vi "Get SMO HELP.vi"(8 "error in (no error)":errorcluster, 10 "Command":string, 11 "Inst.Transport in":refnum<class "Inst.Transport.lvclass">) -> (0 "error out":errorcluster, 2 "output cluster":T1, 3 "Inst.Transport out":refnum<class "Inst.Transport.lvclass">)   [LabVIEW 2019, in "Inst.Transport.lvclass"]
uses:
  Inst.Transport.lvclass
  <userlib>/LevyLab/Instrument Framework/subsystems/Help/typedefs/Help--cluster.ctl
  Typedefs/Inst.Transport.PublicCommands--Enum.ctl
  Typedefs/startTransport--Request--Cluster.ctl
  Typedefs/Inst.Transport.Methods--Enum.ctl
  Typedefs/getStatus--Reply--Cluster.ctl
  Typedefs/Inst.Transport.Status--Enum.ctl
  Typedefs/setExptFolder--Request--Cluster.ctl
  Typedefs/setExptComments--Request--Cluster.ctl
  Typedefs/setExptParam--Request--Cluster.ctl
  <userlib>/LevyLab/LV-Data/LV-Data/Typedefs/Dictionary--cluster.ctl
  Typedefs/setSweepConfig--Request--Cluster.ctl
  <userlib>/LevyLab/Lockin-Multichannel/Instrument.DAQ/Typedefs/Sweep.Channel--Cluster--Array.ctl
  <userlib>/LevyLab/Lockin-Multichannel/Instrument.DAQ/Typedefs/Sweep.Channel--Cluster.ctl
  <userlib>/LevyLab/Lockin-Multichannel/Instrument.DAQ/Typedefs/Sweep.Pattern--Enum.ctl
  <userlib>/LevyLab/Instrument Framework/Instrument Types/SCPI/Instrument.SCPI.lvclass
  <userlib>/LevyLab/Instrument Framework/subsystems/Help/Help.lvclass
  <userlib>/LevyLab/LV-Data/LV-Data/LV-Data.lvclass
  <userlib>/LevyLab/Lockin-Multichannel/Instrument.DAQ/Instrument.DAQ.lvclass
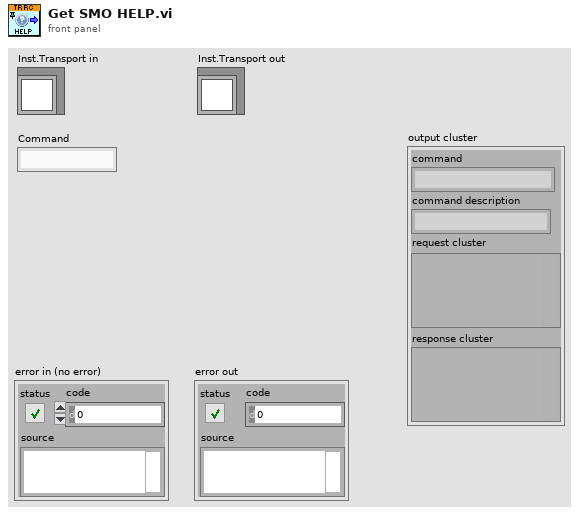
[diagram p1: front panel]
types:
  T1 = typedef "Instrument.lvlib/Help.lvclass/Help--cluster.ctl" = cluster{"command":string, "command description":string, "request cluster":variant, "response cluster":variant}
  T2 = typedef "Inst.Transport.lvclass/Inst.Transport.PublicCommands--Enum.ctl" = enum16{"startTransport", "stopTransport", "getStatus", "setExptFolder", "setExptComments", "appendExptParam", "clearExptParam", "setExptParam", "setSweepConfig"}
  T3 = typedef "Inst.Transport.lvclass/startTransport--Request--Cluster.ctl" = cluster{"method":T4}
  T4 = typedef "Inst.Transport.lvclass/Inst.Transport.Methods--Enum.ctl" = enum16{"LockinSweep", "LockinTime", "LockinTimeDelay"}
  T5 = typedef "Inst.Transport.lvclass/getStatus--Reply--Cluster.ctl" = cluster{"Status":T6}
  T6 = typedef "Inst.Transport.lvclass/Inst.Transport.Status--Enum.ctl" = enum16{"idle", "running"}
  T7 = typedef "Inst.Transport.lvclass/setExptFolder--Request--Cluster.ctl" = cluster{"folder":string}
  T8 = typedef "Inst.Transport.lvclass/setExptComments--Request--Cluster.ctl" = cluster{"comments":string}
  T9 = typedef "Inst.Transport.lvclass/setExptParam--Request--Cluster.ctl" = cluster{"param":T10}
  T10 = typedef "LV-Data.lvclass/Dictionary--cluster.ctl" = cluster{"key":string, "value":variant}
  T11 = typedef "Inst.Transport.lvclass/setSweepConfig--Request--Cluster.ctl" = cluster{"sweepTime":dbl, "initialWaitTime":dbl, "returnToStart":bool, "sweepChannels":T12}
  T12 = typedef "Instrument.Lockin.lvlib/Instrument.DAQ.lvclass/Sweep.Channel--Cluster--Array.ctl" = T13[]
  T13 = typedef "Instrument.Lockin.lvlib/Instrument.DAQ.lvclass/Sweep.Channel--Cluster.ctl" = cluster{"Enable?":bool, "Channel":u16, "Start":dbl, "End":dbl, "Pattern":T14, "Table":dbl[]}
  T14 = typedef "Instrument.Lockin.lvlib/Instrument.DAQ.lvclass/Sweep.Pattern--Enum.ctl" = enum16{"Ramp /", "Ramp /\\", "Smooth Ramp _/", "Smooth Ramp _/\\_", "Table"}
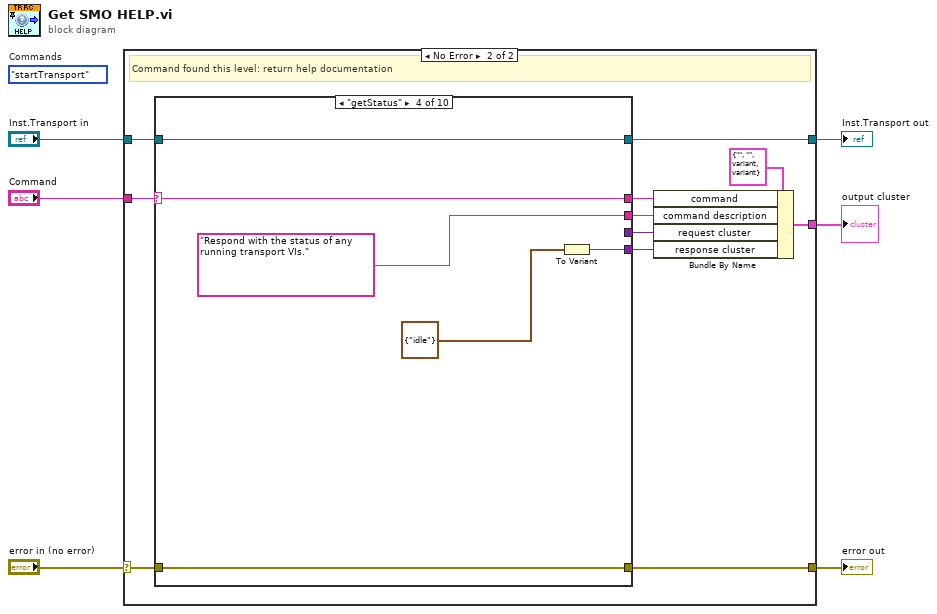
[diagram p0: block diagram]
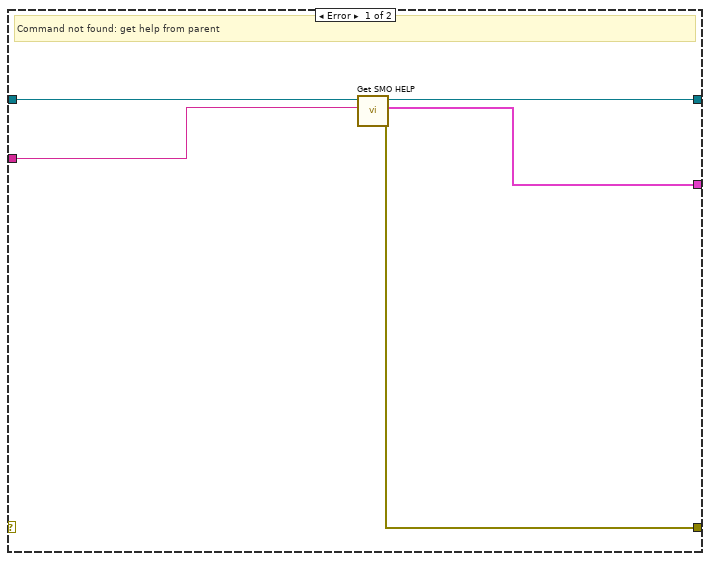
[diagram p2: hidden frame]
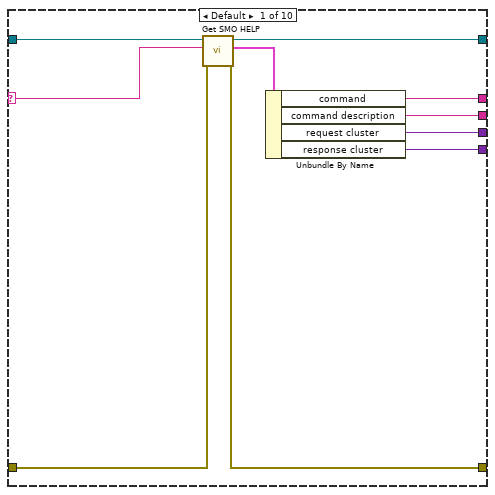
[diagram p3: hidden frame]
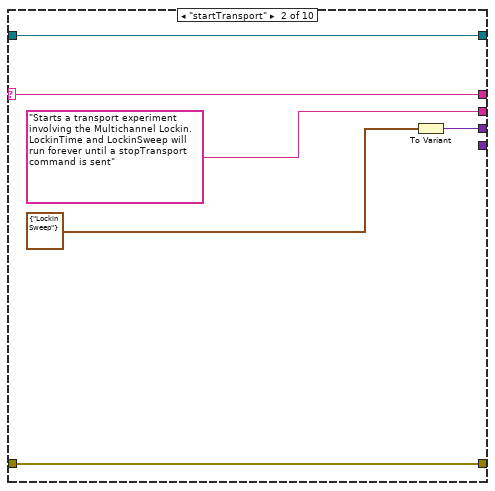
[diagram p4: hidden frame]
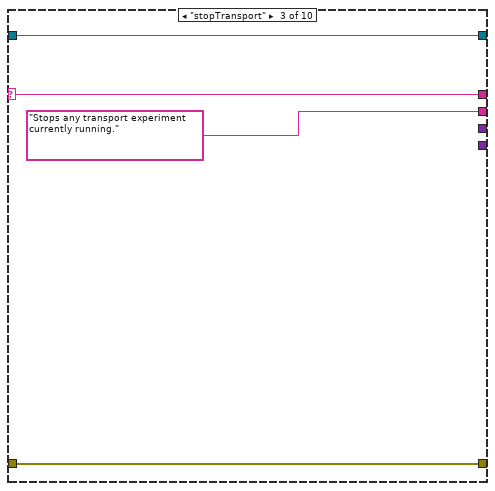
[diagram p5: hidden frame]
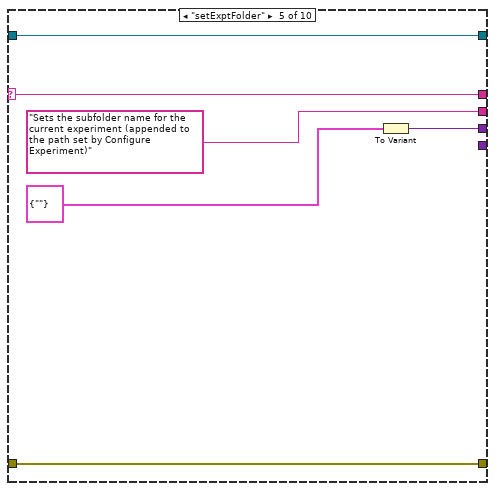
[diagram p6: hidden frame]
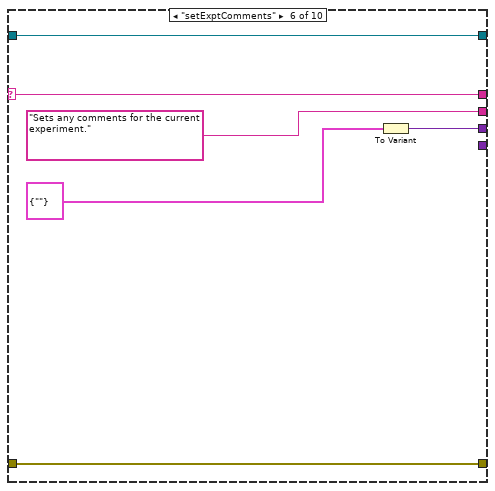
[diagram p7: hidden frame]
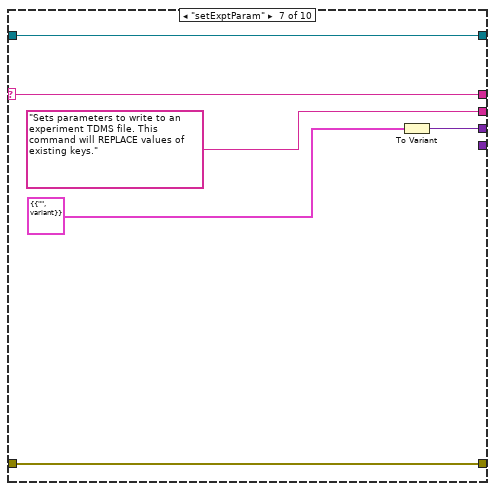
[diagram p8: hidden frame]
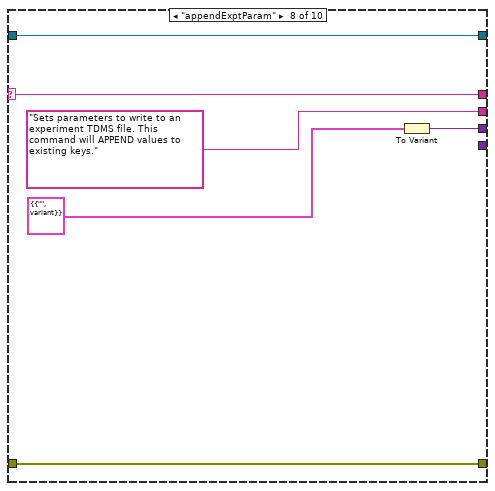
[diagram p9: hidden frame]
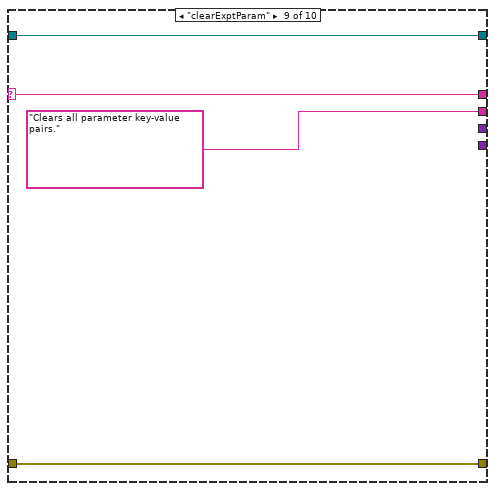
[diagram p10: hidden frame]
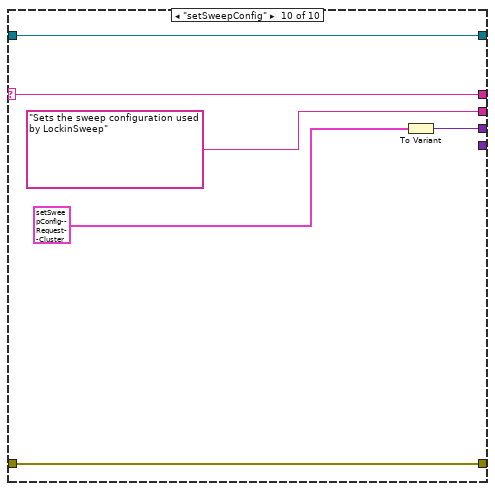
[diagram p11: hidden frame]
diagram:
  (unwired) Inst.Transport.PublicCommands--Enum."startTransport"  # Commands
  n1 = case shown="No Error" "error in (no error)" {
    selector: "error in (no error)" -> [_ w18]
    tunnel: "Inst.Transport in" -> [w11 w13]
    tunnel: [w10 w12] -> w5
    tunnel: [w8 w17] -> w6
    tunnel: [w7 w22] -> w1
    tunnel: "Command" -> [w9 w20]
    frame Error {
      # "Command not found: get help from parent"
      n2 = call-parent "Get SMO HELP.vi"("Command"=w9, "Instrument in"=w11) -> ("error out"=w8:errorcluster, "help cluster"=w7:T1, "Instrument out"=w10:refnum<class "Inst.Transport.lvclass">)  [unwired: 7 in]
    }
    frame No Error {
      # "Command found this level: return help documentation"
      n3 = case shown="\"getStatus\"" w20 {
        selector: w20 -> [w29 w38 w42 w47 w54 w60 w66 w72 w76 w82]
        tunnel: [w27 w38 w42 w47 w54 w60 w66 w72 w76 w82] -> w19
        tunnel: w18 -> [w30 w37 w41 w48 w53 w59 w65 w71 w75 w81]
        tunnel: [w28 w37 w41 w48 w53 w59 w65 w71 w75 w81] -> w17
        tunnel: [w26 "Starts a transport experiment involving the Multichannel Lockin. LockinTime and LockinSweep will run forever until a stopTransport command is sent" "Stops any transport experiment currently running." "Respond with the status of any running transport VIs." "Sets the subfolder name for the current experiment (appended to the path set by Configure Experiment)" "Sets any comments for the current experiment." "Sets parameters to write to an experiment TDMS file. This command will REPLACE values of existing keys." "Sets parameters to write to an experiment TDMS file. This command will APPEND values to existing keys." "Clears all parameter key-value pairs." "Sets the sweep configuration used by LockinSweep"] -> w16
        tunnel: [w25 w33 _ _ w49 w56 w61 w67 _ w77] -> w15
        tunnel: [w24 _ _ w43 _ _ _ _ _ _] -> w14
        tunnel: w13 -> [w32 w35 w39 w45 w51 w57 w63 w69 w73 w79]
        tunnel: [w31 w35 w39 w45 w51 w57 w63 w69 w73 w79] -> w12
        frame Default {
          n4 = call-parent "Get SMO HELP.vi"("error in (no error)"=w30, "Command"=w29, "Instrument in"=w32) -> ("error out"=w28:errorcluster, "help cluster"=w23:T1, "Instrument out"=w31:refnum<class "Inst.Transport.lvclass">)  [unwired: 6 in]
          n5 = Unbundle By Name(w23) -> ("command"=w27:string, "command description"=w26:string, "request cluster"=w25:variant, "response cluster"=w24:variant)
        }
        frame "startTransport" {
          n6 = To Variant(anything=T3 {"method"=enum."LockinSweep"} ("startTransport")) -> (Variant=w33:variant)
        }
        frame "stopTransport" {
        }
        frame "getStatus" {
          n7 = To Variant(anything=T5 {"Status"=enum."idle"} ("getStatus")) -> (Variant=w43:variant)
        }
        frame "setExptFolder" {
          n8 = To Variant(anything=T7 {"folder"=""} ("setExptFolder")) -> (Variant=w49:variant)
        }
        frame "setExptComments" {
          n9 = To Variant(anything=T8 {"comments"=""} ("setExptComments")) -> (Variant=w56:variant)
        }
        frame "setExptParam" {
          n10 = To Variant(anything=T9 {"param"={"key"="", "value"=variant}} ("setExptParam")) -> (Variant=w61:variant)
        }
        frame "appendExptParam" {
          n11 = To Variant(anything=T9 {"param"={"key"="", "value"=variant}} ("setExptParam")) -> (Variant=w67:variant)
        }
        frame "clearExptParam" {
        }
        frame "setSweepConfig" {
          n12 = To Variant(anything=T11 {"sweepTime"=0.0, "initialWaitTime"=0.0, "returnToStart"=FALSE, "sweepChannels"=[{"Enable?"=FALSE, "Channel"=0, "Start"=0.0, "End"=0.1, "Pattern"=enum."Ramp /", "Table"=[1.0]}]} ("setSweepConfig")) -> (Variant=w77:variant)
        }
      }
      n13 = Bundle By Name(cluster=T1 {"command"="", "command description"="", "request cluster"=variant, "response cluster"=variant} ("Help"), "command"=w19, "command description"=w16, "request cluster"=w15, "response cluster"=w14) -> (w22:T1)
    }
  }
  "Inst.Transport out" <- w5
  "output cluster" <- w1
  "error out" <- w6
